vi "Equal.vi"(4 "value case matching (sensitive)":T1=enum."system", 5 "key case matching (sensitive)":T1=enum."system", 6 "array B":T2, 7 "array A":T2) -> (1 "A == B":bool, 2 "duplicate array B":T2, 3 "duplicate array A":T2)   [LabVIEW 2015, in "Car Wash.lvlib" / "Tools_KeyedArray.lvlib"]
doc: "Compares two keyed arrays. You can specify the case sensitivity of the comparison of both the element keys and element values."
uses:
  Tools_KeyedArray.lvlib
  String/Tools_String.lvlib
  KeyedArray.ctl
  <vilib>/FTP/util/Case Matching.ctl
  <vilib>/FTP/NI_FTP.lvlib
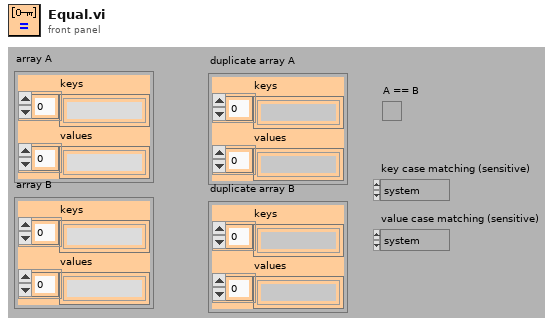
[diagram p1: front panel]
types:
  T1 = typedef "NI_FTP.lvlib/Case Matching.ctl" = enum16{"a != A", "a == A", "system"}
  T2 = typedef "Car Wash.lvlib/Tools_KeyedArray.lvlib/KeyedArray.ctl" = cluster{"keys":string[], "values":string[]}
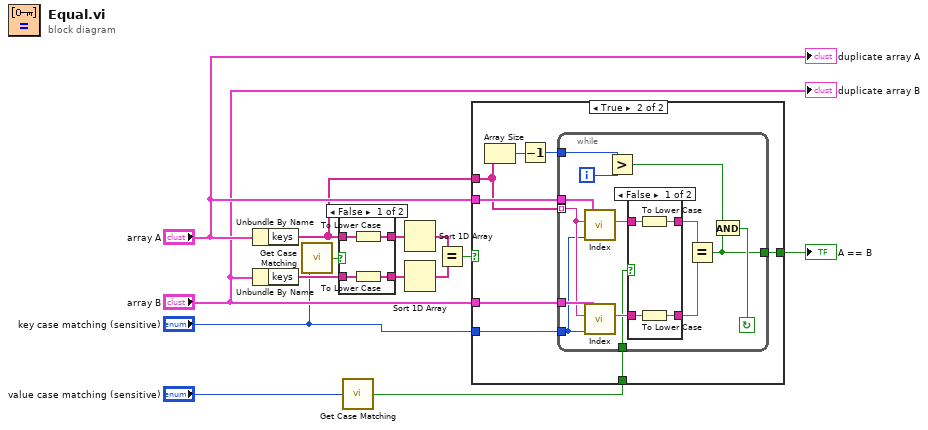
[diagram p0: block diagram]
diagram:
  n1 = Unbundle By Name("array A") -> ("keys"=w5:string[])
  n2 = Unbundle By Name("array B") -> ("keys"=w4:string[])
  n3 = call "Get Case Matching.vi"("string matching"="key case matching (sensitive)") -> ("match case"=w6:bool)
  n4 = case shown="False" w6 {
    tunnel: w5 -> [w18 w20]
    tunnel: w4 -> [w17 w19]
    tunnel: [w16 w20] -> w3
    tunnel: [w15 w19] -> w2
    frame False {
      n5 = To Lower Case(string=w18) -> (all lower case string=w16:string[])
      n6 = To Lower Case(string=w17) -> (all lower case string=w15:string[])
    }
    frame True {
    }
  }
  n7 = call "Get Case Matching.vi"("string matching"="value case matching (sensitive)") -> ("match case"=w7:bool)
  n8 = Sort 1D Array(array=w3) -> (sorted array=w14:string[])
  n9 = Sort 1D Array(array=w2) -> (sorted array=w13:string[])
  n10 = Equal?(x=w14, y=w13) -> (x = y?=w12:bool)
  n11 = case shown="True" w12 {
    selector: w12 -> [w21 _]
    tunnel: "array A" -> [_ w29]
    tunnel: "array B" -> [_ w28]
    tunnel: [w21 w25] -> w9
    tunnel: w7 -> [_ w24]
    tunnel: w5 -> [_ w23]
    tunnel: "key case matching (sensitive)" -> [_ w22]
    frame False {
    }
    frame True {
      n12 = Array Size(array=w23) -> (size(s)=w27:i32)
      n13 = Decrement(x=w27) -> (x-1=w26:i32)
      n14 = while {
        tunnel: w22 -> [w30]
        tunnel: w24 -> [w31]
        tunnel: [w32] -> w25
        tunnel: w26 -> [w36]
        tunnel: w28 -> [w42]
        tunnel: w29 -> [w43]
        tunnel: w23 -> [w41] mode=indexing
        i -> [w35]
        stop <- w33 continue-if-true
        n15 = call "Index.vi"("case matching (sensitive)"=w30, "key"=w41, "array in"=w43) -> ("value"=w40:string)  [unwired: 1 in, 3 out]
        n16 = call "Index.vi"("case matching (sensitive)"=w30, "key"=w41, "array in"=w42) -> ("value"=w38:string)  [unwired: 1 in, 3 out]
        n17 = Greater?(x=w36, y=w35) -> (0:w34:bool)
        n18 = case shown="False" w31 {
          tunnel: w40 -> [w45 w49]
          tunnel: [w44 w49] -> w39
          tunnel: w38 -> [w47 w48]
          tunnel: [w46 w48] -> w37
          frame False {
            n19 = To Lower Case(string=w45) -> (all lower case string=w44:string)
            n20 = To Lower Case(string=w47) -> (all lower case string=w46:string)
          }
          frame True {
          }
        }
        n21 = Equal?(x=w39, y=w37) -> (x = y?=w32:bool)
        n22 = And(x=w34, y=w32) -> (x .and. y?=w33:bool)
      }
    }
  }
  "A == B" <- w9
  "duplicate array A" <- "array A"
  "duplicate array B" <- "array B"
